vi "Read Correct params.vi"(8 "error in (no error)":errorcluster, 11 "Data in":refnum<class "CV-Main.lvclass">) -> (0 "error out":errorcluster, 2 "Correct params":refnum<data-value>, 3 "Data out":refnum<class "CV-Main.lvclass">)   [LabVIEW 2013, in "CameraVision.lvlib" / "CV-Main.lvclass"]
uses:
  CV-Main.lvclass
  Correction/CV-Correction.lvclass
  CV-Main.lvclass/CV-Main.ctl
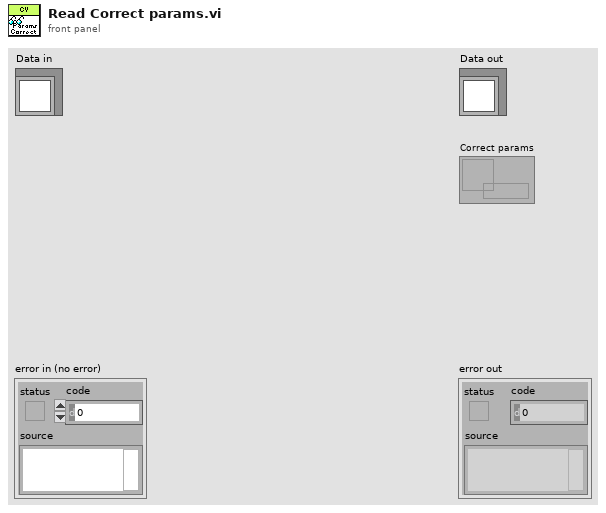
[diagram p1: front panel]
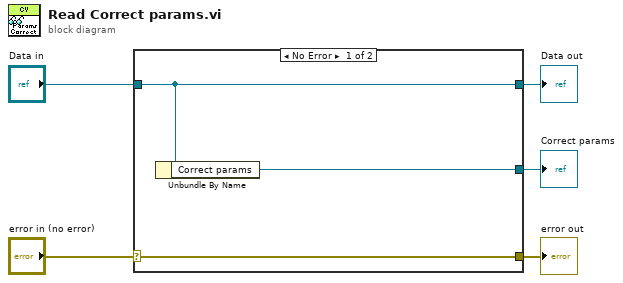
[diagram p0: block diagram]
diagram:
  n1 = case shown="No Error" "error in (no error)" {
    selector: "error in (no error)" -> [w8 w9]
    tunnel: [w8 w9] -> w4
    tunnel: [w7 w10] -> w2
    tunnel: "Data in" -> [w7 w10]
    tunnel: [w6 _] -> w1
    frame No Error {
      n2 = Unbundle By Name(w7) -> ("Correct params"=w6:refnum<data-value>)
    }
    frame Error {
    }
  }
  "error out" <- w4
  "Data out" <- w2
  "Correct params" <- w1
